vi "BinaryToDecimal.vi"(1 "Unsigned?":bool, 2 "Binary":bool[](array[boolean]), 3 "Inverse?":bool=TRUE) -> (0 "Decimal":dbl)   [LabVIEW 2013]
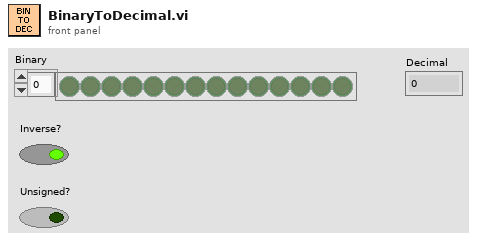
[diagram p1: front panel]
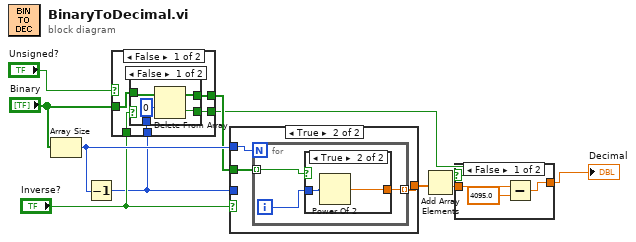
[diagram p0: block diagram]
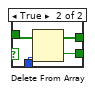
[diagram p3: hidden frame]
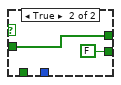
[diagram p4: hidden frame]
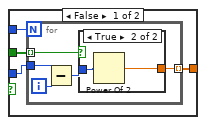
[diagram p5: hidden frame]
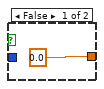
[diagram p6: hidden frame]
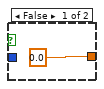
[diagram p7: hidden frame]
diagram:
  n1 = Array Size(array="Binary") -> (size(s)=w9:i32)
  n2 = Decrement(x=w9) -> (x-1=w4:i32)
  n3 = case shown="False" "Unsigned?" {
    tunnel: "Binary" -> [w13 w25]
    tunnel: [w12 w25] -> w7
    tunnel: "Inverse?" -> [w15 _]
    tunnel: w4 -> [w14 _]
    tunnel: [w11 FALSE ("Boolean")] -> w1
    frame False {
      n4 = case shown="False" w15 {
        tunnel: w14 -> [_ w22]
        tunnel: w13 -> [w19 w23]
        tunnel: [w17 w21] -> w12
        tunnel: [w16 w20] -> w11
        frame False {
          n5 = Delete From Array(array=w19, index=0) -> (deleted portion=w16:bool, array with subset deleted=w17:bool[])  [unwired: 1 in]
        }
        frame True {
          n6 = Delete From Array(array=w23, index=w22) -> (deleted portion=w20:bool, array with subset deleted=w21:bool[])  [unwired: 1 in]
        }
      }
    }
    frame True {
    }
  }
  n7 = case shown="True" "Inverse?" {
    tunnel: w7 -> [w29 w40]
    tunnel: [w28 w39] -> w10
    tunnel: w9 -> [w27 w38]
    tunnel: w4 -> [w26 _]
    frame False {
      n8 = for {
        N: w27 -> [_]
        tunnel: w29 -> [w34] mode=indexing
        tunnel: [w33] -> w28 mode=indexing
        tunnel: w26 -> [w31]
        i -> [w32]
        n9 = Subtract(x=w31, y=w32) -> (x-y=w30:i32)
        n10 = case shown="True" w34 {
          tunnel: w30 -> [_ w37]
          tunnel: [0.0 w36] -> w33
          frame False {
          }
          frame True {
            n11 = Power Of 2(x=w37) -> (2^x=w36:dbl)
          }
        }
      }
    }
    frame True {
      n12 = for {
        N: w38 -> [_]
        tunnel: [w43] -> w39 mode=indexing
        tunnel: w40 -> [w41] mode=indexing
        i -> [w42]
        n13 = case shown="True" w41 {
          tunnel: w42 -> [_ w46]
          tunnel: [0.0 w45] -> w43
          frame False {
          }
          frame True {
            n14 = Power Of 2(x=w46) -> (2^x=w45:dbl)
          }
        }
      }
    }
  }
  n15 = Add Array Elements(numeric array=w10) -> (sum=w2:dbl)
  n16 = case shown="False" w1 {
    tunnel: [w47 w50] -> w3
    tunnel: w2 -> [w49 w50]
    frame False {
      n17 = Subtract(x=w49, y=4095.0) -> (x-y=w47:dbl)
    }
    frame True {
    }
  }
  "Decimal" <- w3
